vi "Actual Sample Mode [SM] Core.vi"(8 "error in (no error)":errorcluster, 11 "CS++Scope":refnum<class "CS++Scope.lvclass">) -> (0 "error out":errorcluster, 2 "sample mode":i32, 3 "CS++Scope out":refnum<class "CS++Scope.lvclass">)   [LabVIEW 2015, in "CS++Scope.lvlib" / "CS++Scope.lvclass"]
doc: "This VI returns the sample mode the oscilloscope is currently using."
uses:
  CS++Scope.lvclass
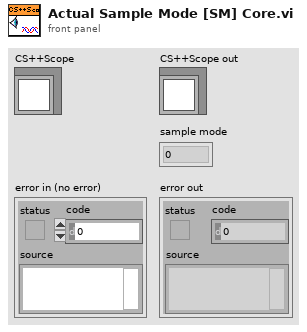
[diagram p1: front panel]
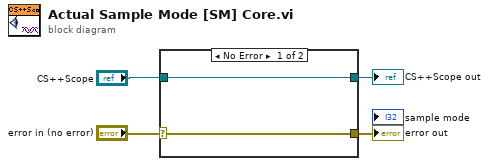
[diagram p0: block diagram]
diagram:
  n1 = case shown="No Error" "error in (no error)" {
    selector: "error in (no error)" -> [w5 w8]
    tunnel: [w5 w8] -> w3
    tunnel: [w6 w7] -> w1
    tunnel: "CS++Scope" -> [w6 w7]
    frame No Error {
    }
    frame Error {
    }
  }
  "error out" <- w3
  "CS++Scope out" <- w1
